vi "LS350Monitor.vi"() -> ()   [LabVIEW 2019]
uses:
  Utility/Monitor Communication/LS350/LS350-cluster.ctl
  Global/Global Variables/Data_Display_global.vi
  Equipment/Lake Shore 350/Lake Shore 350.lvlib
panel:
  in  "stop":bool
  in  "Lakeshore 350":T1 {"Setpoint control" format="%6_5f"}
  out "error out":errorcluster
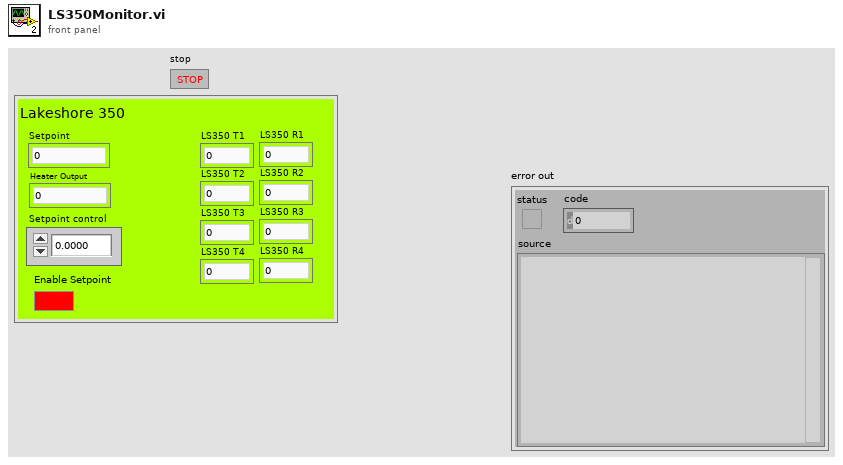
[diagram p1: front panel]
types:
  T1 = typedef "LS350-cluster.ctl" = cluster{"Setpoint":dbl, "Heater Output":dbl, "Setpoint control":dbl, "Enable Setpoint":bool, "LS350 T1":dbl, "LS350 T2":dbl, "LS350 T3":dbl, "LS350 T4":dbl, "LS350 R1":dbl, "LS350 R2":dbl, "LS350 R3":dbl, "LS350 R4":dbl}
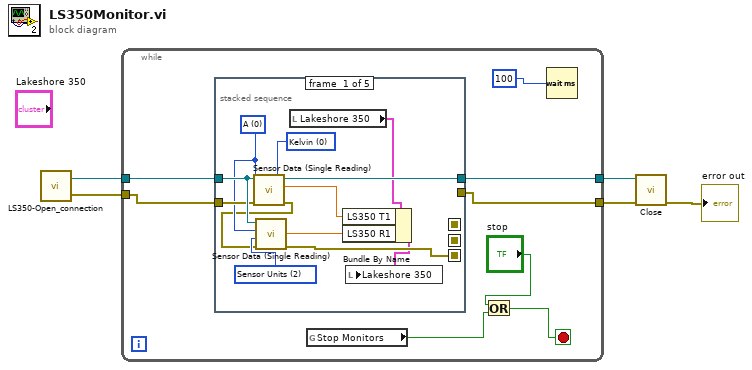
[diagram p0: block diagram]
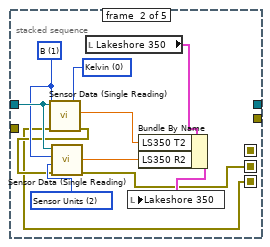
[diagram p2: hidden frame]
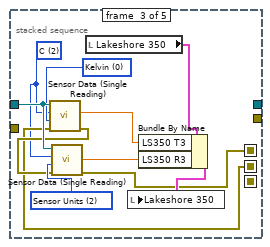
[diagram p3: hidden frame]
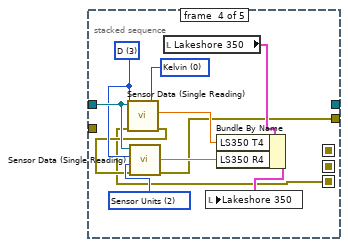
[diagram p4: hidden frame]
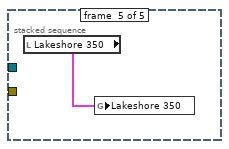
[diagram p5: hidden frame]
diagram:
  n1 = call "LS350-Open_connection.vi"() -> ("error out"=w2:errorcluster, "VISA resource name out"=w3:refnum<visa-resource-name>)  [unwired: 2 in]
  n2 = while {
    tunnel: [w11] -> w5
    tunnel: [w9] -> w4
    tunnel: w3 -> [w13]
    tunnel: w2 -> [w12]
    stop <- w6 stop-if-true
    n3 = stacked-sequence {
      seq-local: [w15 _ _ _ _] -> [_ w27 _ w49 _]
      seq-local: [_ w26 _ _ _] -> [_ _ w39 _ _]
      seq-local: [_ _ w38 _ _] -> [_ _ _ _ _]
      tunnel: w13 -> [w24 w36 w47 w58 _]
      tunnel: w12 -> [w23 _ _ _ _]
      tunnel: [w25 _ _ _ _] -> w11
      tunnel: [_ _ _ w48 _] -> w9
      frame #0 {
        w20 = u16 2 items=["Kelvin", "Celsius", "Sensor Units"] ("Data Source (0:Kelvin)")
        w22 = u16 0 items=["Kelvin", "Celsius", "Sensor Units"] ("Data Source (0:Kelvin)")
        w21 = u16 0 items=["A", "B", "C", "D", "D2", "D3", "D4", "D5"] ("Input (0:A)")
        n4 = call "Sensor Data (Single Reading).vi"("error in (no error)"=w23, "Data Source (0:Kelvin)"=w22, "Input (0:A)"=w21, "VISA resource name"=w24) -> ("error out"=w16:errorcluster, "Sensor Data"=w17:dbl, "VISA resource name out"=w25:refnum<visa-resource-name>)  [unwired: 5 in]
        n5 = call "Sensor Data (Single Reading).vi"("error in (no error)"=w16, "Data Source (0:Kelvin)"=w20, "Input (0:A)"=w21, "VISA resource name"=w24) -> ("error out"=w15:errorcluster, "Sensor Data"=w18:dbl)  [unwired: 5 in, 1 out]
        n6 = local read "Lakeshore 350"() -> (w19:T1)
        n7 = Bundle By Name(cluster=w19, "LS350 T1"=w17, "LS350 R1"=w18) -> (w14:T1)
        n8 = local write "Lakeshore 350"(w14) -> ()
      }
      frame #1 {
        w33 = u16 2 items=["Kelvin", "Celsius", "Sensor Units"] ("Data Source (0:Kelvin)")
        w35 = u16 0 items=["Kelvin", "Celsius", "Sensor Units"] ("Data Source (0:Kelvin)")
        w34 = u16 1 items=["A", "B", "C", "D", "D2", "D3", "D4", "D5"] ("Input (0:A)")
        n9 = call "Sensor Data (Single Reading).vi"("error in (no error)"=w27, "Data Source (0:Kelvin)"=w35, "Input (0:A)"=w34, "VISA resource name"=w36) -> ("error out"=w29:errorcluster, "Sensor Data"=w30:dbl)  [unwired: 5 in, 1 out]
        n10 = call "Sensor Data (Single Reading).vi"("error in (no error)"=w29, "Data Source (0:Kelvin)"=w33, "Input (0:A)"=w34, "VISA resource name"=w36) -> ("error out"=w26:errorcluster, "Sensor Data"=w31:dbl)  [unwired: 5 in, 1 out]
        n11 = local read "Lakeshore 350"() -> (w32:T1)
        n12 = Bundle By Name(cluster=w32, "LS350 T2"=w30, "LS350 R2"=w31) -> (w28:T1)
        n13 = local write "Lakeshore 350"(w28) -> ()
      }
      frame #2 {
        w45 = u16 2 items=["Kelvin", "Celsius", "Sensor Units"] ("Data Source (0:Kelvin)")
        w46 = u16 0 items=["Kelvin", "Celsius", "Sensor Units"] ("Data Source (0:Kelvin)")
        w37 = u16 2 items=["A", "B", "C", "D", "D2", "D3", "D4", "D5"] ("Input (0:A)")
        n14 = call "Sensor Data (Single Reading).vi"("error in (no error)"=w39, "Data Source (0:Kelvin)"=w46, "Input (0:A)"=w37, "VISA resource name"=w47) -> ("error out"=w41:errorcluster, "Sensor Data"=w42:dbl)  [unwired: 5 in, 1 out]
        n15 = call "Sensor Data (Single Reading).vi"("error in (no error)"=w41, "Data Source (0:Kelvin)"=w45, "Input (0:A)"=w37, "VISA resource name"=w47) -> ("error out"=w38:errorcluster, "Sensor Data"=w43:dbl)  [unwired: 5 in, 1 out]
        n16 = local read "Lakeshore 350"() -> (w44:T1)
        n17 = Bundle By Name(cluster=w44, "LS350 T3"=w42, "LS350 R3"=w43) -> (w40:T1)
        n18 = local write "Lakeshore 350"(w40) -> ()
      }
      frame #3 {
        w55 = u16 2 items=["Kelvin", "Celsius", "Sensor Units"] ("Data Source (0:Kelvin)")
        w57 = u16 0 items=["Kelvin", "Celsius", "Sensor Units"] ("Data Source (0:Kelvin)")
        w56 = u16 3 items=["A", "B", "C", "D", "D2", "D3", "D4", "D5"] ("Input (0:A)")
        n19 = call "Sensor Data (Single Reading).vi"("error in (no error)"=w49, "Data Source (0:Kelvin)"=w57, "Input (0:A)"=w56, "VISA resource name"=w58) -> ("error out"=w51:errorcluster, "Sensor Data"=w52:dbl)  [unwired: 5 in, 1 out]
        n20 = call "Sensor Data (Single Reading).vi"("error in (no error)"=w51, "Data Source (0:Kelvin)"=w55, "Input (0:A)"=w56, "VISA resource name"=w58) -> ("error out"=w48:errorcluster, "Sensor Data"=w53:dbl)  [unwired: 5 in, 1 out]
        n21 = local read "Lakeshore 350"() -> (w54:T1)
        n22 = Bundle By Name(cluster=w54, "LS350 T4"=w52, "LS350 R4"=w53) -> (w50:T1)
        n23 = local write "Lakeshore 350"(w50) -> ()
      }
      frame #4 {
        n24 = local read "Lakeshore 350"() -> (w59:T1)
        n25 = global write "Data_Display_global.vi" "Lakeshore 350"(w59) -> ()
      }
    }
    n26 = global read "Data_Display_global.vi" "Stop Monitors"() -> (w7:bool)
    n27 = Or(x="stop", y=w7) -> (x .or. y?=w6:bool)
    n28 = Wait (ms)(milliseconds to wait=100) -> ()  [unwired: 1 out]
  }
  n29 = call "Close.vi"("error in (no error)"=w4, "VISA resource name"=w5) -> ("error out"=→"error out":errorcluster)  [unwired: 9 in]
